vi "Find All Callers of State.vi"(8 "error in (no error)":errorcluster, 9 "State Name":string, 10 "Category (Optional)":string, 11 "JKI SM in":refnum<class "JKI SM.lvclass">) -> (0 "error out":errorcluster, 2 "Callers":T1(array[cluster]), 3 "JKI SM out":refnum<class "JKI SM.lvclass">)   [LabVIEW 2013, in "JKI State Machine API.lvlib" / "JKI SM.lvclass"]
uses:
  JKI SM.lvclass
  <vilib>/Utility/traverseref.llb/TRef TravTarget.ctl
  JKI SM.lvclass/JKI SM.ctl
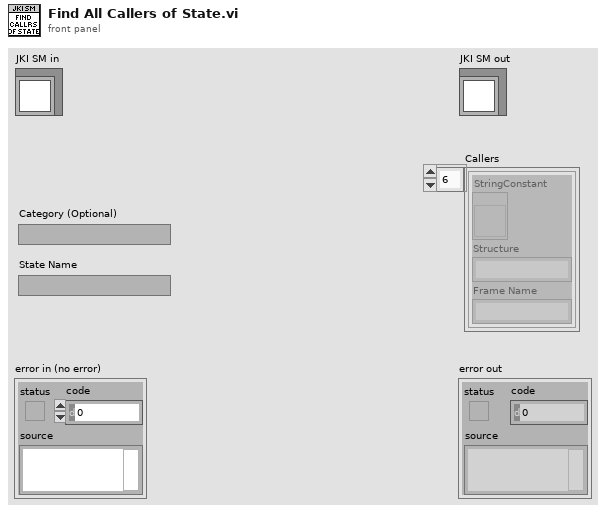
[diagram p1: front panel]
types:
  T1 = cluster{"StringConstant":refnum<vi>, "Structure":string, "Frame Name":string}[]
  T2 = typedef "TRef TravTarget.ctl" = enum16{"FP", "BD", "Other"}
  T3 = cluster{"StringConstant":refnum<vi>, "Structure":string, "Frame Name":string}
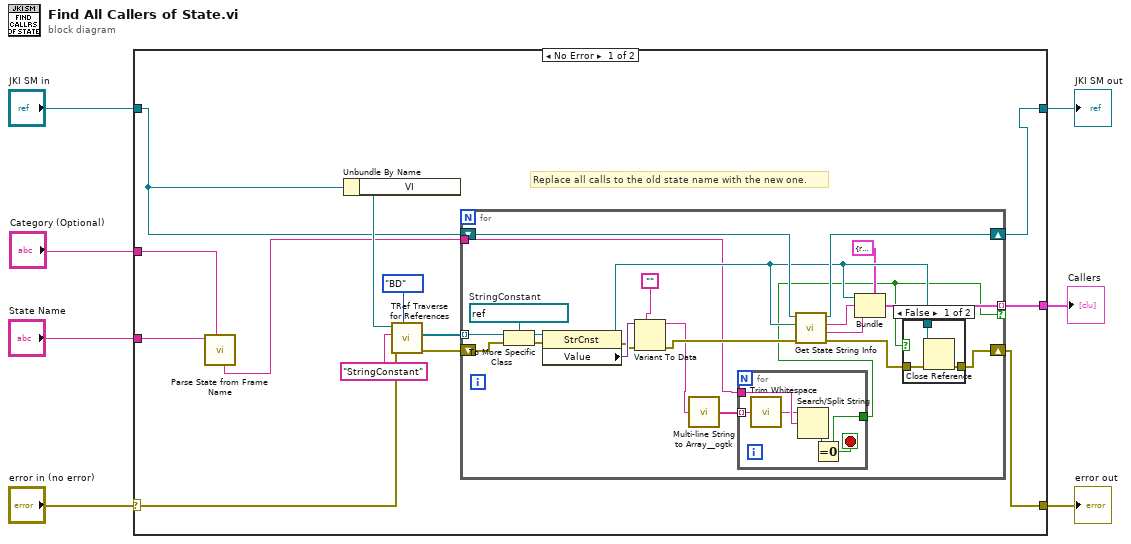
[diagram p0: block diagram]
diagram:
  n1 = case shown="No Error" "error in (no error)" {
    selector: "error in (no error)" -> [w12 w53]
    tunnel: [w11 w53] -> w6
    tunnel: [w13 w52] -> w4
    tunnel: "JKI SM in" -> [w14 w52]
    tunnel: "State Name" -> [w20 _]
    tunnel: "Category (Optional)" -> [w8 _]
    tunnel: [w10 _] -> w1
    frame No Error {
      # "Replace all calls to the old state name with the new one."
      n2 = call "Parse State from Frame Name.vi"("Category (Optional)"=w8, "Frame or State Name"=w20) -> ("\"Category: State\" String"=w9:string)  [unwired: 5 in, 4 out]
      n3 = Unbundle By Name(w14) -> ("VI"=w15:refnum<vi>)
      n4 = call <vilib>:"TRef Traverse for References.vi"("Traverse Target"=TRef_TravTarget."BD", "error in (no error)"=w12, "Class Name"="StringConstant", "VI Refnum"=w15) -> ("error out"=w16:errorcluster, "References"=w17:refnum<vi>[])  [unwired: 1 in, 5 out]
      n5 = for {
        tunnel: w17 -> [w42] mode=indexing
        tunnel: w9 -> [w22]
        shift-right: [w32] -> w13
        shift-left: w14 -> [w31]
        shift-right: [w30] -> w11
        shift-left: w16 -> [w39]
        tunnel: [w27] -> w10 mode=indexing if=w21
        w40 = refnum<vi> refnum  # StringConstant
        n6 = To More Specific Class(target class=w40, reference=w42, error in=w39) -> (specific class reference=w41:refnum<vi>, error out=w38:errorcluster)
        n7 = property class="StrCnst"(reference=w41, error in=w38) -> (reference out=w29:refnum<vi>, error out=w34:errorcluster, "Value"=w37:variant)
        n8 = Variant To Data(error in=w34, type="", Variant=w37) -> (data=w24:string, error out=w35:errorcluster)
        n9 = call <userlib>:"Multi-line String to Array__ogtk.vi"("string"=w24) -> ("lines"=w23:string[])
        n10 = for {
          tunnel: w23 -> [w47] mode=indexing
          tunnel: w22 -> [w46]
          tunnel: [w43] -> w21
          stop <- w43 stop-if-true
          n11 = call <vilib>:"Trim Whitespace.vi"("string"=w47) -> ("trimmed string"=w45:string)  [unwired: 1 in]
          n12 = Search/Split String(string=w45, search string/char (-)=w46) -> (offset of match=w44:i32)  [unwired: 1 in, 2 out]
          n13 = Equal To 0?(x=w44) -> (x = 0?=w43:bool)
        }
        n14 = call "Get State String Info.vi"("error in (no error)"=w35, "StrCnst Refnum in"=w29, "JKI SM in"=w31) -> ("error out"=w33:errorcluster, "Frame Name"=w25:string, "Structure"=w28:string, "JKI SM out"=w32:refnum<class "JKI SM.lvclass">)  [unwired: 5 in]
        n15 = Bundle(cluster=T3 {"StringConstant"=refnum, "Structure"="", "Frame Name"=""}, "StringConstant"=w29, "Structure"=w28, "Frame Name"=w25) -> (w27:T3)
        n16 = case shown="False" w21 {
          tunnel: w33 -> [w50 w51]
          tunnel: [w49 w51] -> w30
          tunnel: w29 -> [w48 _]
          frame False {
            n17 = Close Reference(reference=w48, error in (no error)=w50) -> (error out=w49:errorcluster)
          }
          frame True {
          }
        }
      }
    }
    frame Error {
    }
  }
  "error out" <- w6
  "JKI SM out" <- w4
  "Callers" <- w1
